vi "Read Invocation Request ID.vi"(8 "error in (no error)":errorcluster, 11 "Invocation Request in":refnum<class "Invocation Request ID.lvclass">) -> (0 "error out":errorcluster, 2 "Invocation Request ID":u64, 3 "Invocation Request out":refnum<class "Invocation Request ID.lvclass">)   [LabVIEW 2021, in "wamplv.lvlib" / "Invocation Request ID.lvclass"]
uses:
  Invocation Request ID.lvclass
  Invocation Request ID.lvclass/Invocation Request ID.ctl
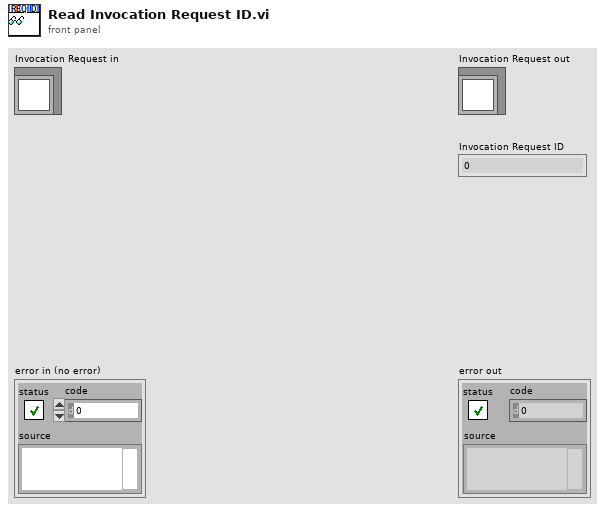
[diagram p1: front panel]
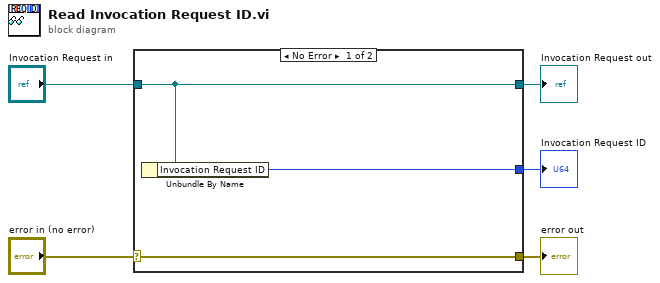
[diagram p0: block diagram]
diagram:
  n1 = case shown="No Error" "error in (no error)" {
    selector: "error in (no error)" -> [w8 w9]
    tunnel: [w8 w9] -> w4
    tunnel: [w7 w10] -> w2
    tunnel: "Invocation Request in" -> [w7 w10]
    tunnel: [w6 _] -> w1
    frame No Error {
      n2 = Unbundle By Name(w7) -> ("Invocation Request ID"=w6:u64)
    }
    frame Error {
    }
  }
  "error out" <- w4
  "Invocation Request out" <- w2
  "Invocation Request ID" <- w1
